vi "Target Field Rate (Read).vi"(6 "ISOBUS address":T3=-1 caption="ISOBUS address (-1)", 8 "error in":errorcluster, 11 "Mercury Reference In":T4) -> (0 "error out":errorcluster, 1 "Unit":T1, 2 "Target Field Rate":dbl, 3 "Mercury Reference Out":T4, 4 "Valid?":T2)   [LabVIEW 2015, in "Mercury iXX.lvlib" / "Magnet.lvlib"]
doc: "Acquire the most recent target field rate reading."
uses:
  Magnet.lvlib
  Controls/Mercury Reference.ctl
  Controls/Comms Transport Layer.ctl
  private/Controls/Query Dynamic Reference.ctl
  Controls/ISOBus Address.ctl
  Controls/Is Valid LED.ctl
  Controls/Unit String.ctl
  private/Controls/Command Verbs.ctl
  Mercury iXX.lvlib
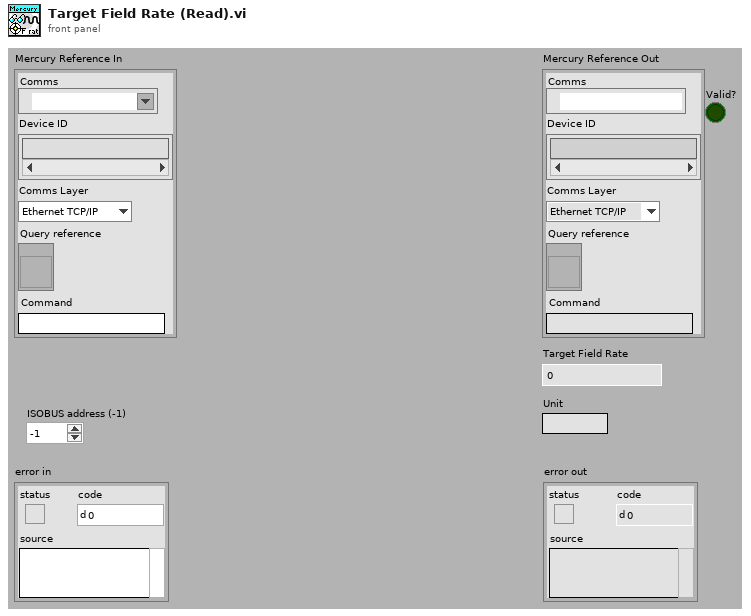
[diagram p1: front panel]
types:
  T1 = typedef "Mercury iXX.lvlib/Unit String.ctl" = string
  T2 = typedef "Mercury iXX.lvlib/Is Valid LED.ctl" = bool
  T3 = typedef "Mercury iXX.lvlib/ISOBus Address.ctl" = i32
  T4 = typedef "Mercury iXX.lvlib/Mercury Reference.ctl" = cluster{"Comms":refnum<visa-resource-name>, "Device ID":string[], "Comms Layer":T5, "Command":string, "Query reference":T6}
  T5 = typedef "Mercury iXX.lvlib/Comms Transport Layer.ctl" = enum16{"Ethernet TCP/IP", "USB", "ISOBus - RS-232", "GPIB"}
  T6 = typedef "Mercury iXX.lvlib/Query Dynamic Reference.ctl" = refnum<vi>
  T7 = typedef "Mercury iXX.lvlib/Command Verbs.ctl" = string
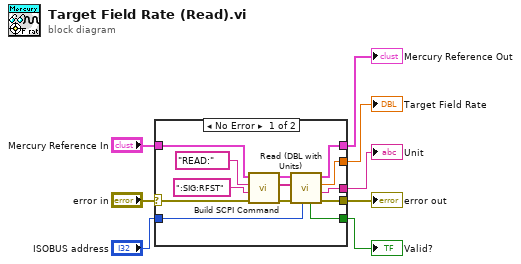
[diagram p0: block diagram]
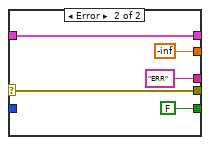
[diagram p2: hidden frame]
diagram:
  n1 = case shown="No Error" "error in" {
    selector: "error in" -> [w10 w25]
    tunnel: "ISOBUS address" -> [w21 _]
    tunnel: [w20 T2 FALSE ("Valid?")] -> w7
    tunnel: [w19 w25] -> w6
    tunnel: [w18 T1 "ERR" ("Unit")] -> w5
    tunnel: [w17 w26] -> w4
    tunnel: [w16 -inf] -> w3
    tunnel: "Mercury Reference In" -> [w13 w26]
    frame No Error {
      n2 = call "Build SCPI Command.vi"("error in"=w10, "Noun(s)"=":SIG:RFST" ("Command"), "Verb"=T7 "READ:", "Mercury Reference In"=w13) -> ("error out"=w11:errorcluster, "SCPI Message(s)"=w9:string[], "Mercury Reference Out"=w12:T4)  [unwired: 5 out]
      n3 = call "Read (DBL with Units).vi"("ISOBUS address"=w21, "error in"=w11, "SCPI Message(s)"=w9, "Mercury Reference In"=w12) -> ("error out"=w19:errorcluster, "Unit"=w18:T1, "Data (Dbl)"=w16:dbl, "Mercury Reference Out"=w17:T4, "Valid?"=w20:T2)  [unwired: 3 out]
    }
    frame Error {
    }
  }
  "Mercury Reference Out" <- w4
  "error out" <- w6
  "Valid?" <- w7
  "Unit" <- w5
  "Target Field Rate" <- w3
